vi "Open.vi"(8 "Error In":errorcluster, 10 "Remote Path":string, 11 "SFTP":refnum<class "SFTP.lvclass">) -> (0 "Error Out":errorcluster, 3 "SFTP Directory":refnum<class "SFTP Directory.lvclass">)   [LabVIEW 2018, in "Toolkit.lvlib" / "SFTP Directory.lvclass"]
uses:
  SFTP Directory.lvclass
  SFTP/SFTP.lvclass
  SFTP/SFTP.lvclass/SFTP.ctl
  SFTP Directory.lvclass/SFTP Directory.ctl
  Toolkit.lvlib
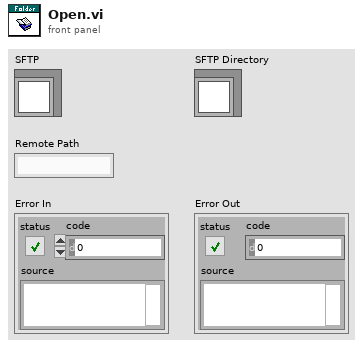
[diagram p1: front panel]
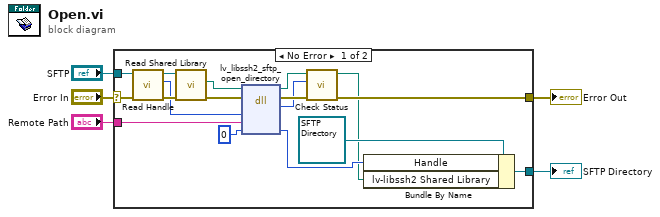
[diagram p0: block diagram]
diagram:
  n1 = case shown="No Error" "Error In" {
    selector: "Error In" -> [w16 w23]
    tunnel: [w10 w23] -> w4
    tunnel: "SFTP" -> [w17 _]
    tunnel: "Remote Path" -> [w22 _]
    tunnel: [w6 _] -> w1
    frame No Error {
      n2 = call "Read Handle.vi"("Error In"=w16, "SFTP In"=w17) -> ("Erorr Out"=w14:errorcluster, "Handle"=w12:u64, "SFTP Out"=w15:refnum<class "SFTP.lvclass">)  [unwired: 7 in]
      n3 = call "Read Shared Library.vi"("Error In"=w14, "SFTP In"=w15) -> ("Erorr Out"=w11:errorcluster, "lv-libssh2 Shared Library"=w13:path)  [unwired: 7 in, 1 out]
      n4 = dll-call lib="lv-libssh2.*" fn="lv_libssh2_sftp_open_directory"(path in=w13, error in=w11, "sftp"=w12, "path"=w22, "handle"=u64 0) -> (path out=w21:path, error out=w20:errorcluster, "status"=w19:i32, "handle"=w8:u64)  [unwired: 3 in]
      n5 = call "Check Status.vi"("Error In"=w20, "Status"=w19, "lv-libssh2 Shared Library In"=w21) -> ("Error Out"=w10:errorcluster, "lv-libssh2 Shared Library Out"=w7:path)  [unwired: 7 in]
      n6 = Bundle By Name(cluster=refnum<class "SFTP Directory.lvclass"> refnum ("Toolkit.lvlib:SFTP Directory.lvclass"), "Handle"=w8, "lv-libssh2 Shared Library"=w7) -> (w6:refnum<class "SFTP Directory.lvclass">)
    }
    frame Error {
    }
  }
  "Error Out" <- w4
  "SFTP Directory" <- w1
